vi "qp_active set core.vi"(5 "b":dbl[](array[numeric]), 7 "A":T1, 9 "x":dbl[](array[numeric]), 10 "c":dbl[](array[numeric]), 11 "Q":T1) -> (2 "Qx+c":dbl[](array[numeric]), 3 "p_k":dbl[](array[numeric]))   [LabVIEW 2020, in "NI_Gmath.lvlib"]
uses:
  NI_Gmath.lvlib
  RealMatrix.ctl
  A x Vector.vi
  Matrix left divisionMV_general_direct.vi
  NI_AALBase.lvlib
  NI_Matrix.lvlib
panel:
  out "error out":errorcluster
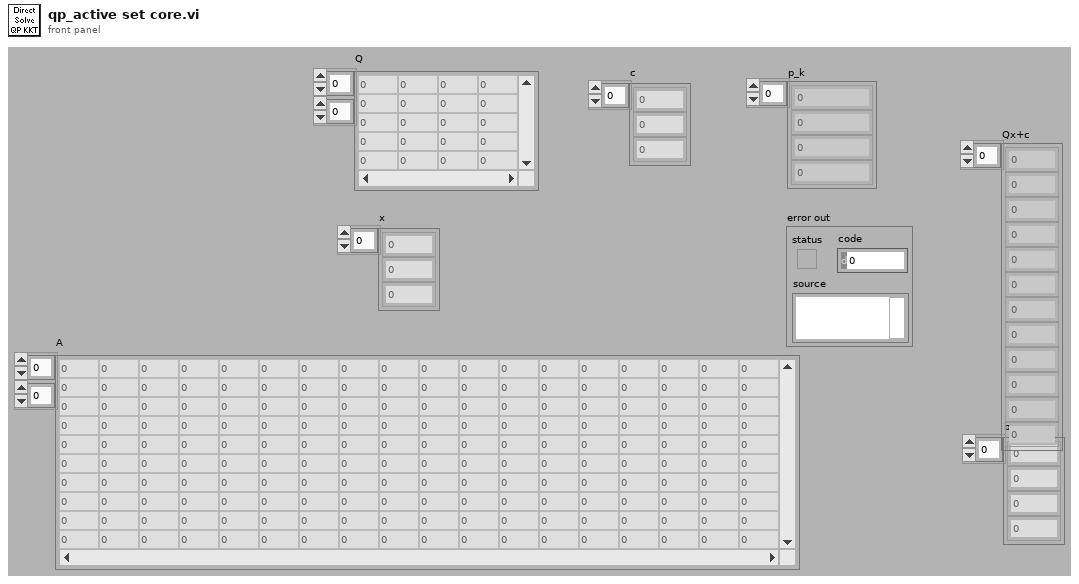
[diagram p1: front panel]
types:
  T1 = typedef "NI_Matrix.lvlib/RealMatrix.ctl" = dbl[][]
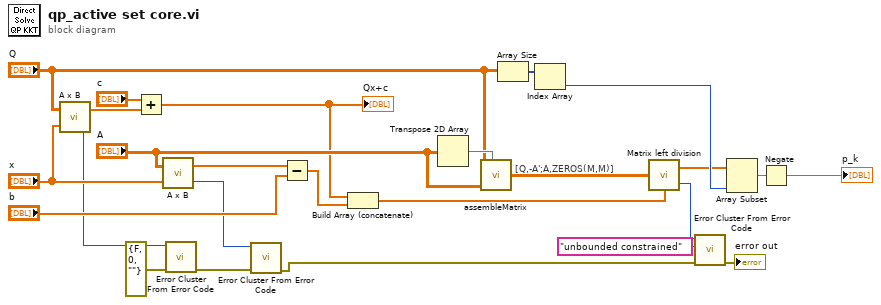
[diagram p0: block diagram]
diagram:
  # "[Q,-A';A,ZEROS(M,M)]"
  n1 = call-poly "A x B.vi"("Vector"="x", "A"="Q") -> ("error"=w5:i32, "A x Vector"=w10:dbl[])
  n2 = Add ("Add.vi")(x="c", y=w10) -> (x+y=w14:dbl[])
  "Qx+c" <- w14
  n3 = call-poly "A x B.vi"("Vector"="x", "A"="A") -> ("error"=w4:i32, "A x Vector"=w15:dbl[])
  n4 = call "Error Cluster From Error Code.vi"("error in (no error)"=errorcluster {"status"=FALSE, "code"=0, "source"=""}, "error code (0)"=w5) -> ("error out"=w3:errorcluster)  [unwired: 7 in]
  n5 = call "Error Cluster From Error Code.vi"("error in (no error)"=w3, "error code (0)"=w4) -> ("error out"=w2:errorcluster)  [unwired: 7 in]
  n6 = Subtract(x=w15, y="b") -> (x-y=w12:dbl[])
  n7 = Build Array (concatenate)(w14, w12) -> (w8:dbl[])
  n8 = Transpose 2D Array(2D array="A") -> (transposed array=w25:T1)
  n9 = call "assembleMatrix.vi"("A"="Q", "B"=w25, "C"="A") -> ("ABCD"=w9:dbl[][])  [unwired: 2 in]
  n10 = Array Size(array="Q") -> (size(s)=w22:i32[])
  n11 = Index Array(array=w22) -> (element=w21:i32)  [unwired: 1 in]
  n12 = call-poly "Matrix left division.vi"("A"=w8, "B"=w9) -> ("error"=w6:i32, "B\\A"=w7:dbl[])  [unwired: 2 in]
  n13 = call "Error Cluster From Error Code.vi"("error in (no error)"=w2, "error message (\"\")"="unbounded constrained" ("error message (\"\")"), "error code (0)"=w6) -> ("error out"=→"error out":errorcluster)  [unwired: 6 in]
  n14 = Array Subset(array=w7, length=w21) -> (w20:dbl[])  [unwired: 1 in]
  n15 = Negate(x=w20) -> (-x=→"p_k":dbl[])
